vi "add_Pose2D.vi"(6 "Pose2D":cluster{"x":dbl, "y":dbl, "theta":dbl}, 7 "msg in":string) -> (3 "msg out":string)   [LabVIEW 2015]
doc: "Flattens a pose 2D into a message"
uses:
  std_msgs/subs/float64Scalar.vi
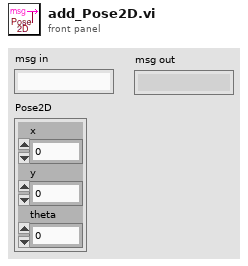
[diagram p1: front panel]
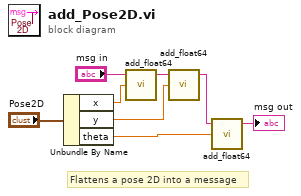
[diagram p0: block diagram]
diagram:
  # "Flattens a pose 2D into a message"
  n1 = Unbundle By Name("Pose2D") -> ("x"=w3:dbl, "y"=w2:dbl, "theta"=w1:dbl)
  n2 = call-poly "add_float64.vi"("Numeric"=w3, "msg in"="msg in") -> ("msg out"=w6:string)  [unwired: 3 in]
  n3 = call-poly "add_float64.vi"("Numeric"=w2, "msg in"=w6) -> ("msg out"=w5:string)  [unwired: 3 in]
  n4 = call-poly "add_float64.vi"("Numeric"=w1, "msg in"=w5) -> ("msg out"=→"msg out":string)  [unwired: 3 in]
